vi "getsteeringangle.vi"(10 "Target Pose":T1, 11 "Current Robot":T1) -> (2 "x-y":dbl)   [LabVIEW 2017]
uses:
  040-typeDefs/Position.ctl
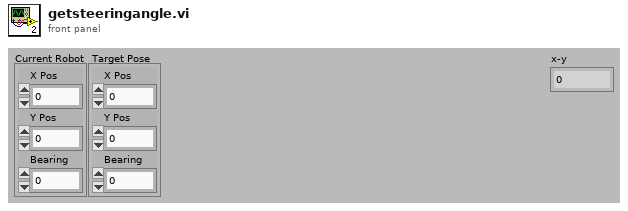
[diagram p1: front panel]
types:
  T1 = typedef "Position.ctl" = cluster{"X Pos":dbl, "Y Pos":dbl, "Bearing":dbl}
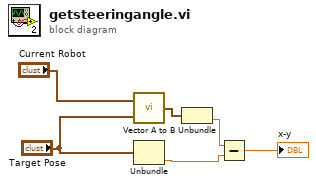
[diagram p0: block diagram]
diagram:
  n1 = call "Vector A to B.vi"("Destination"="Target Pose", "Current"="Current Robot") -> ("vector"=w4:cluster{dbl, "Bearing":dbl})
  n2 = Unbundle("Target Pose") -> ("Bearing"=w2:dbl)  [unwired: 2 out]
  n3 = Unbundle(w4) -> ("Bearing"=w1:dbl)  [unwired: 1 out]
  n4 = Subtract(x=w1, y=w2) -> (x-y=→"x-y":dbl)
